vi "donothing.vi"() -> ()   [LabVIEW 2023]
panel:
  out "Array":string[](array[string])
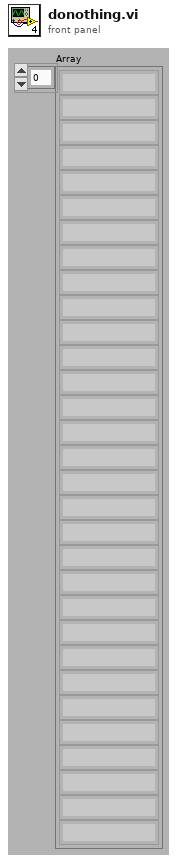
[diagram p1: front panel]
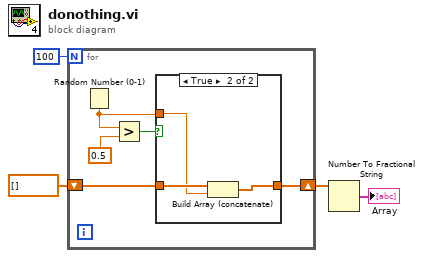
[diagram p0: block diagram]
diagram:
  n1 = for {
    N: 100 -> [_]
    shift-right: [w5] -> w2
    shift-left: dbl[] [] -> [w7]
    n2 = Random Number (0-1)() -> (number: 0 to 1=w6:dbl)
    n3 = Greater?(x=w6, y=0.5) -> (0:w8:bool)
    n4 = case shown="True" w8 {
      tunnel: w7 -> [w10 w13]
      tunnel: w6 -> [_ w12]
      tunnel: [w10 w11] -> w5
      frame False {
      }
      frame True {
        n5 = Build Array (concatenate)(w13, w12) -> (w11:dbl[])
      }
    }
  }
  n6 = Number To Fractional String(number=w2) -> (F-format string=→"Array":string[])  [unwired: 3 in]
